vi "#459.vi"() -> ()   [LabVIEW 2017]
uses:
  user.lib/_NEVSTOP/Communicable State Machine(CSM)/Utility/_support/Periodic String Filter Level.ctl
  user.lib/_NEVSTOP/Communicable State Machine(CSM)/Utility/Periodic String Filter Setting.ctl
  user.lib/_NEVSTOP/Communicable State Machine(CSM)/AdvanceAPI/CSM - Revert Arguments-Safe String.vi
  user.lib/_NEVSTOP/Communicable State Machine(CSM)/_Shared/Trim Single-line Text.vi
  user.lib/_NEVSTOP/Communicable State Machine(CSM)/AdvanceAPI/CSM - Make String Arguments Safe.vi
  user.lib/_NEVSTOP/Communicable State Machine(CSM)/AdvanceAPI/CSM - Break Down Multiple States String.vi
  user.lib/_NEVSTOP/Communicable State Machine(CSM)/AdvanceAPI/CSM - Compact Multiple States.vi
  user.lib/_NEVSTOP/Communicable State Machine(CSM)/AdvanceAPI/CSM - Keywords.vi
  user.lib/_NEVSTOP/Communicable State Machine(CSM)/Communicable State Machine.lvlib
  user.lib/_NEVSTOP/Communicable State Machine(CSM)/addons/Watchdog/CSM Watchdog.lvlib
  user.lib/_NEVSTOP/Communicable State Machine(CSM)/addons/Logger/CSM File Logger.lvlib
  user.lib/_NEVSTOP/Communicable State Machine(CSM)/addons/Logger/CSM File Logger Limit.ctl
panel:
  out "State History 2":string
  in  "Exit":bool
  out "Waveform Chart":dbl(graph)
  out "Since Exiting(s)":dbl format="%.2f"
  out "LogInQ":i32
  out "State History":string
  out "log handling Speed(#/s)":dbl
  out "LogInQ changing Speed(#/s)":dbl
  out "Level":T1
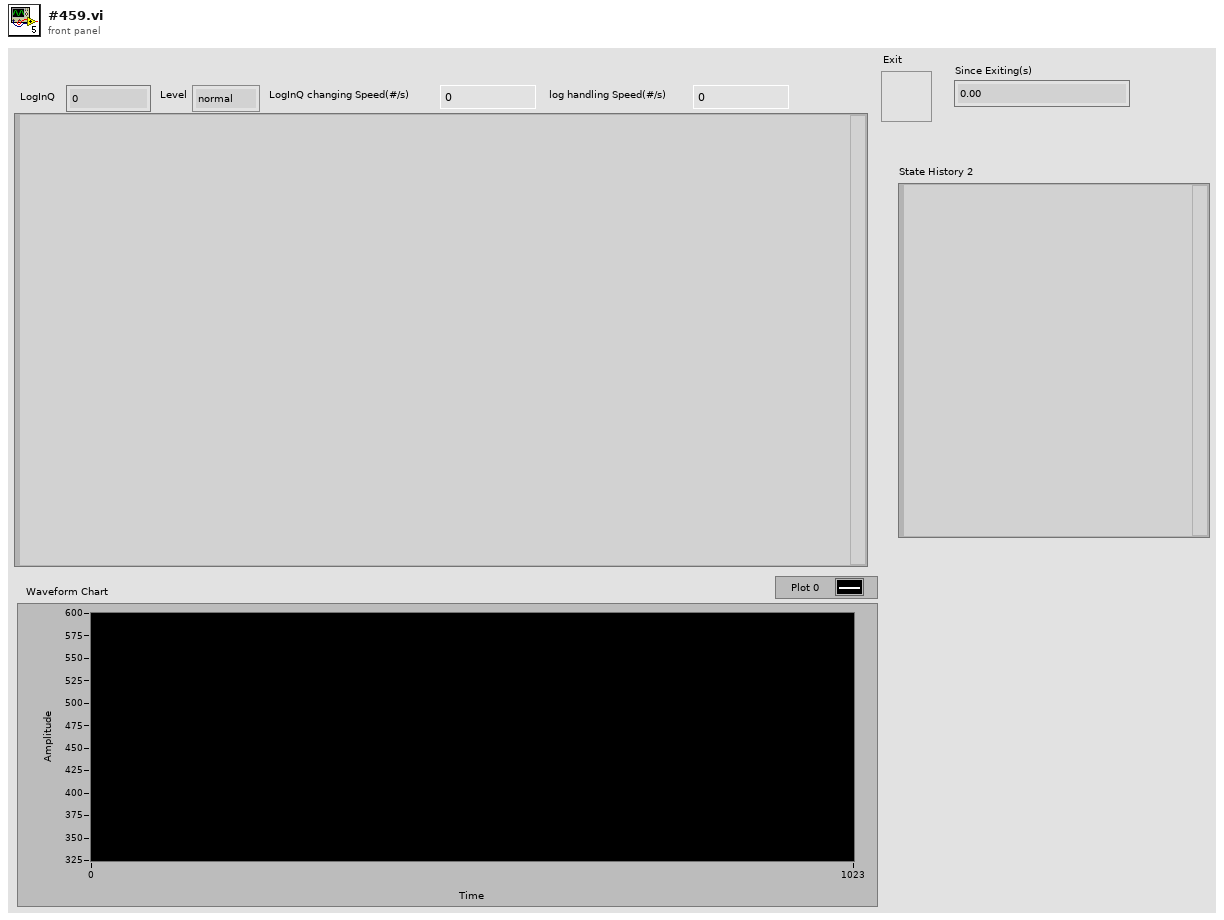
[diagram p1: front panel]
types:
  T1 = typedef "Communicable State Machine.lvlib/Periodic String Filter Level.ctl" = enum16{"normal", "L1", "L2", "L3", "L4"}
  T2 = typedef "CSM File Logger.lvlib/CSM File Logger Limit.ctl" = cluster{"file size (in bytes)":i64, "file num":i32}
  T3 = typedef "Communicable State Machine.lvlib/Periodic String Filter Setting.ctl" = cluster{"threashold(#/s)":dbl, "Check Peroid(s)":dbl}
  T4 = typedef "Communicable State Machine.lvlib/_CSM_GlobalLog_MSG.ctl" = cluster{"Name(\"\" to use uuid)":string, "Current State":string, "Arguments":string, "Source Message":T5, "Source Module":string, "Complete(T)/Start(F)":bool, "LogType":T6, "Time Stamp":timestamp}
  T5 = typedef "Communicable State Machine.lvlib/_CSM_Response Source Message.ctl" = cluster{"‘State":string, "’Arguments":string, "’Error":errorcluster}
  T6 = typedef "Communicable State Machine.lvlib/_CSM_GlobalLog_MSG_TYPE.ctl" = enum16{"User Log", "State Change", "Status", "Interrupt", "Register", "Unregister", "Error Log", "Module Created", "Module Destroyed"}
  T7 = enum32{"Invalid", "Standard", "Closed", "Hidden", "Minimized", "Maximized"}
  T8 = enum32{"invalid app kind", "Development System", "Run Time System", "Student Edition", "Embedded LabVIEW", "Evaluation", "Custom"}
  T9 = cluster{"Current VI Reference":refnum<vi>, "Close Panel on Exit?":bool}
  T10 = cluster{"Core":cluster{"Current VI Reference":refnum<vi>, "Close Panel on Exit?":bool}, "Your Boolean data":bool, "Your string data":string}
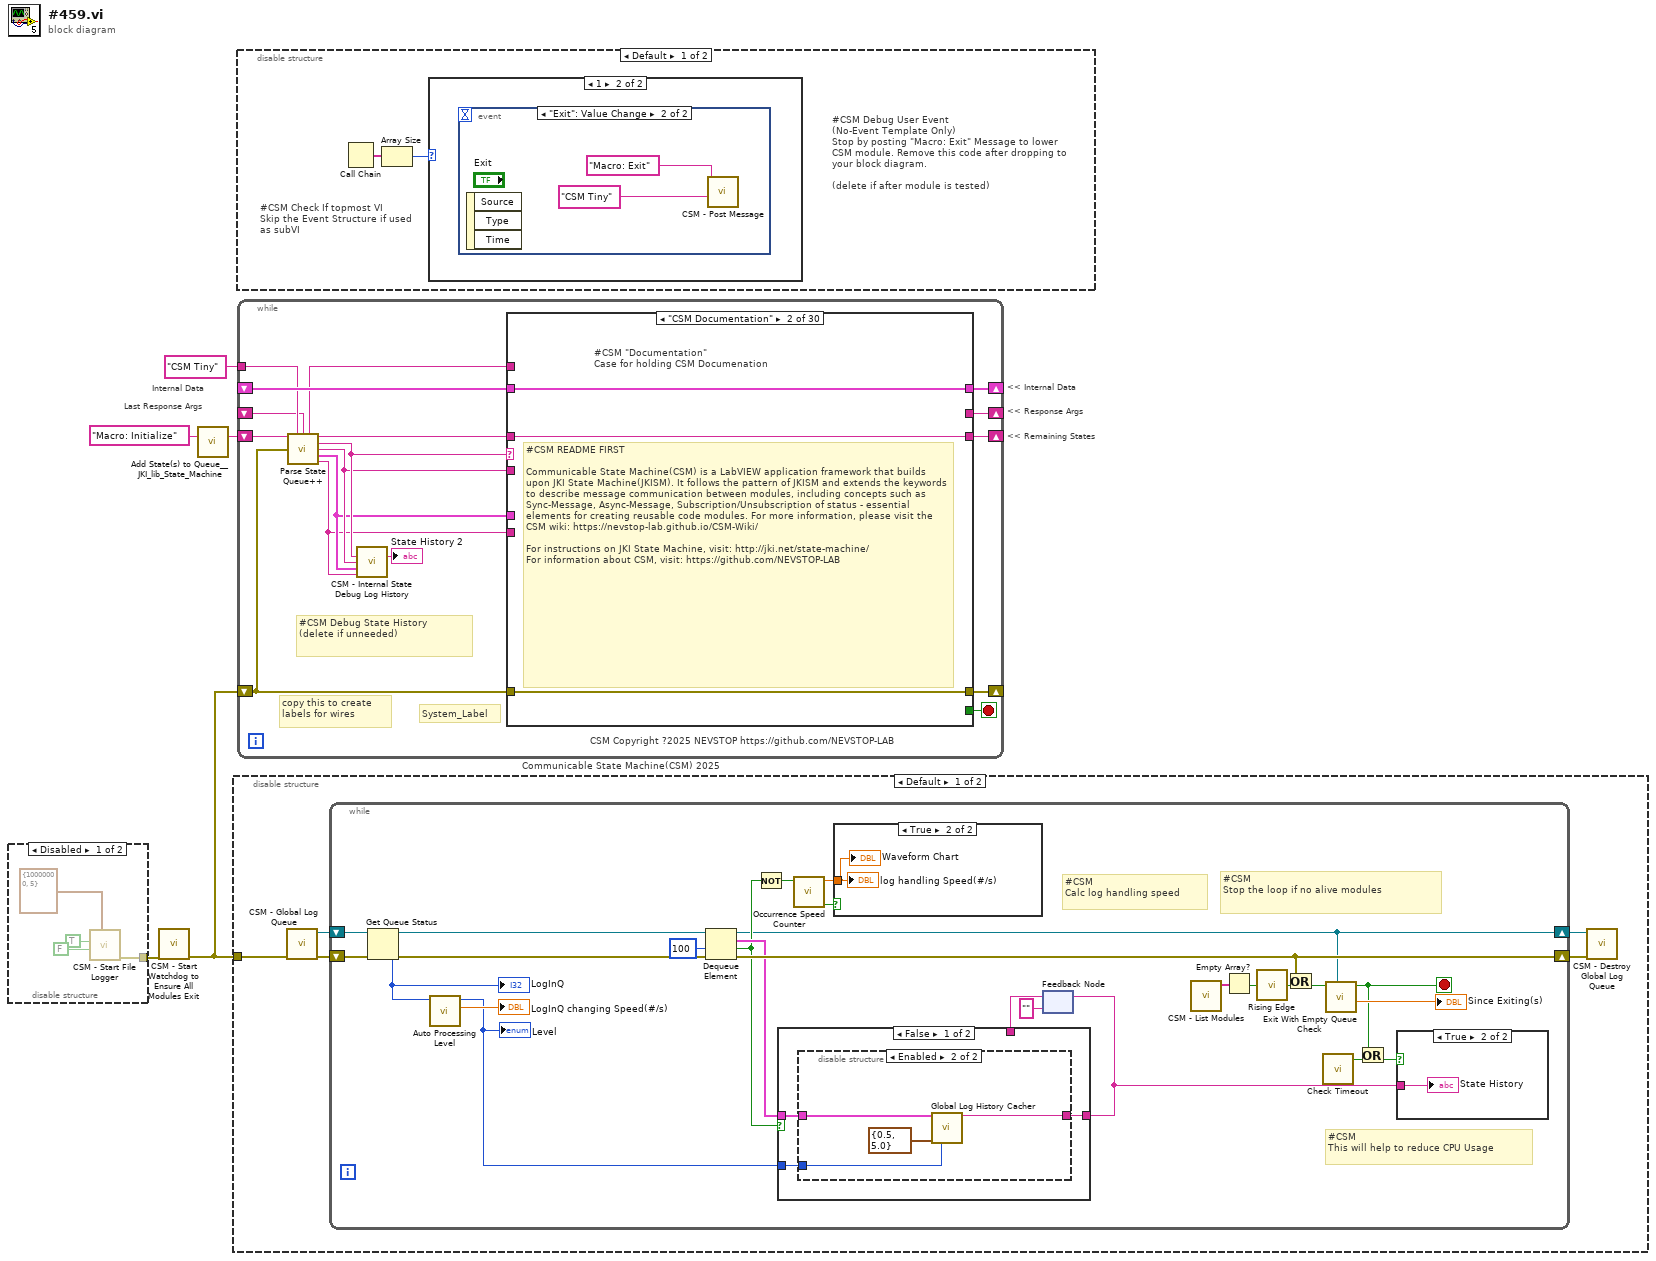
[diagram p0: block diagram]
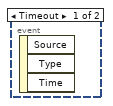
[diagram p3: hidden frame]
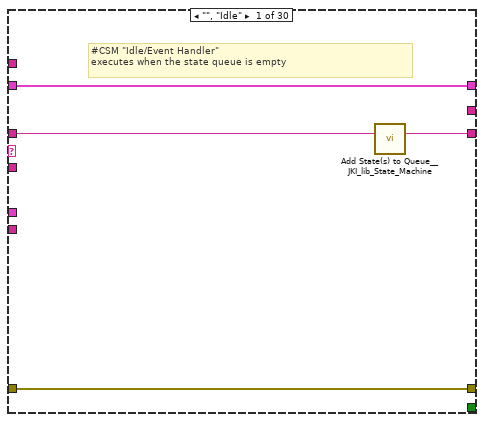
[diagram p5: hidden frame]
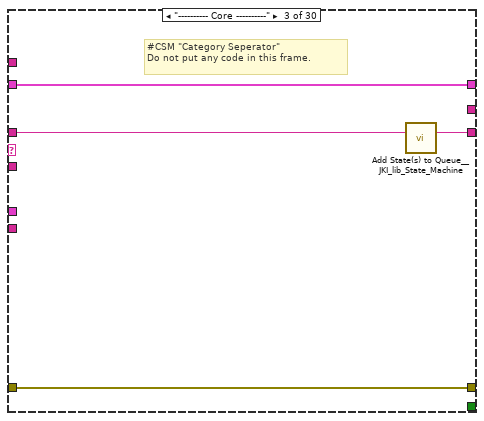
[diagram p6: hidden frame]
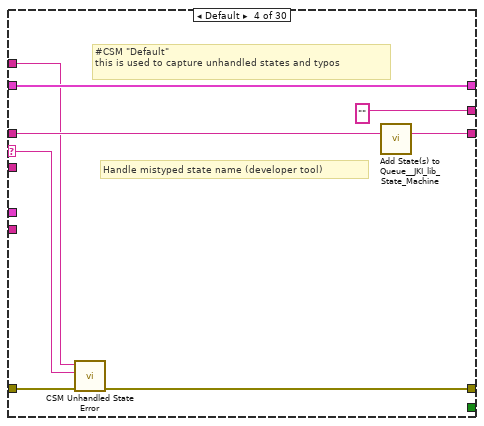
[diagram p7: hidden frame]
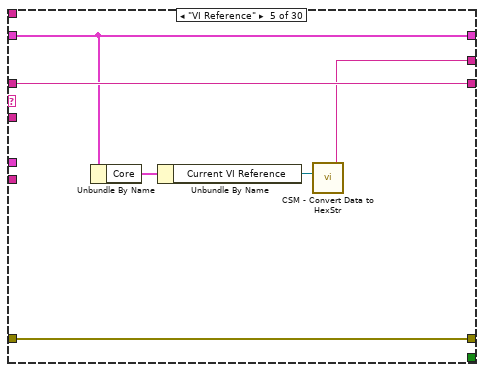
[diagram p8: hidden frame]
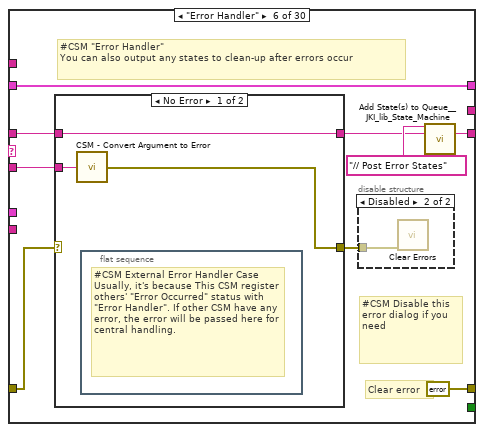
[diagram p9: hidden frame]
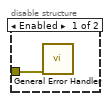
[diagram p10: hidden frame]
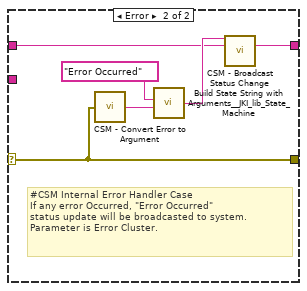
[diagram p11: hidden frame]
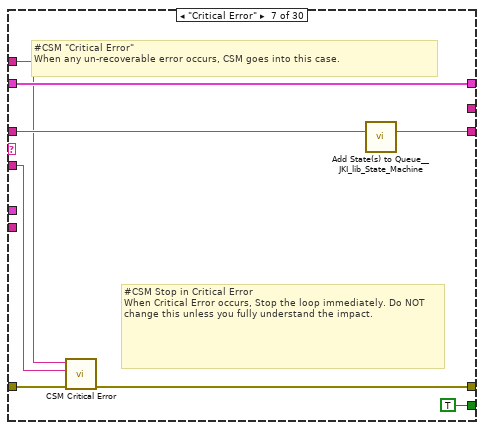
[diagram p12: hidden frame]
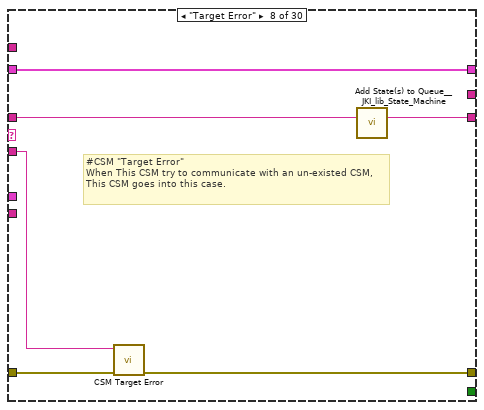
[diagram p13: hidden frame]
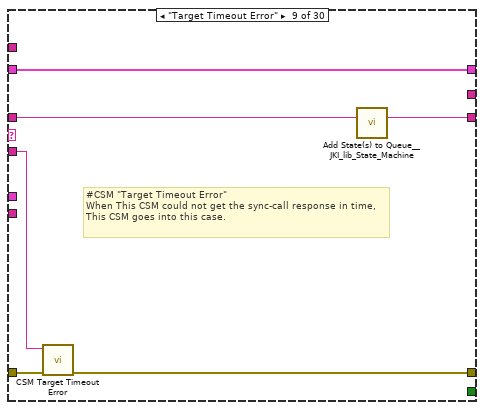
[diagram p14: hidden frame]
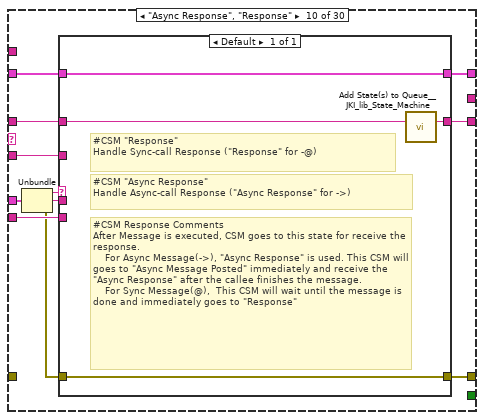
[diagram p15: hidden frame]
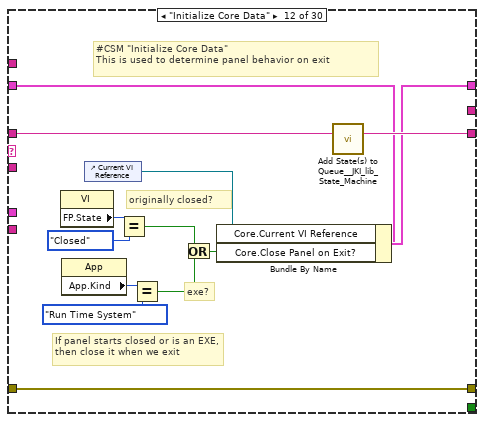
[diagram p17: hidden frame]
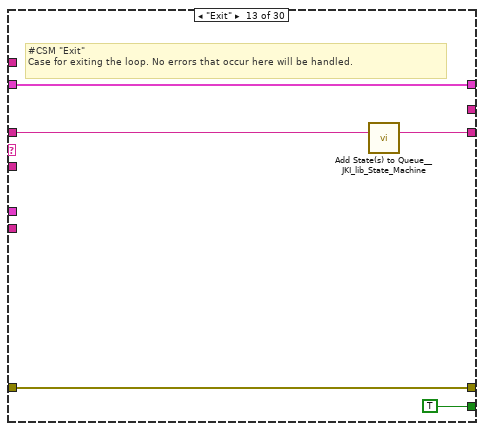
[diagram p18: hidden frame]
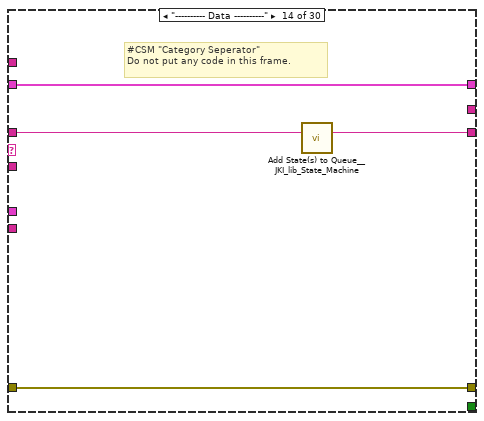
[diagram p19: hidden frame]
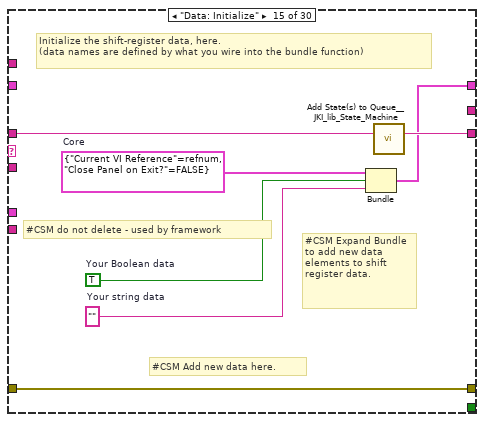
[diagram p20: hidden frame]
diagram:
  # "Last Response Args"
  # "Internal Data"
  # "<< Internal Data"
  # "<< Response Args"
  # "<< Remaining States"
  n1 = disable-structure shown="Disabled" {
    disable-tunnel: [w9 _] -> w5
    frame Disabled {
      n2 = call "CSM - Start File Logger.vi"("log limit"=T2 {"file size (in bytes)"=10000000, "file num"=5}, "WatchDog? (T)"=FALSE, "Exit When All Module Exist?(F)"=TRUE) -> ("Error out"=w9:errorcluster)  [unwired: 6 in, 2 out]
    }
    frame Enabled {
    }
  }
  n3 = call "CSM - Start Watchdog to Ensure All Modules Exit.vi"("error in (no error)"=w5) -> ("error out"=w1:errorcluster)  [unwired: 10 in]
  n4 = call <vilib>:"Add State(s) to Queue__JKI_lib_State_Machine.vi"("State(s) in (\"\")"="Macro: Initialize" ("Init State(\"Macro: Initialize\")")) -> ("States Out"=w2:string)  [unwired: 14 in]
  n5 = disable-structure shown="Default" {
    disable-tunnel: w1 -> [w10 _]
    frame condition #0 (active) {
      n6 = call "CSM - Global Log Queue.vi"("Error in"=w10) -> ("Error out"=w13:errorcluster, "GlobalEvent Queue"=w11:refnum<queue>)  [unwired: 9 in]
      n7 = while {
        shift-right: [w39] -> w14
        shift-left: w13 -> [w36]
        shift-right: [w27] -> w12
        shift-left: w11 -> [w40]
        stop <- w20 stop-if-true
        # "#CSM\nCalc log handling speed"
        # "#CSM\nStop the loop if no alive modules"
        # "#CSM\nThis will help to reduce CPU Usage"
        n8 = Get Queue Status(queue=w40, error in (no error)=w36) -> (queue out=w38:refnum<queue>, error out=w37:errorcluster, # elements in queue=w23:i32)  [unwired: 1 in, 5 out]
        "LogInQ" <- w23
        n9 = call "Auto Processing Level.vi"("#Left In Q"=w23) -> ("LogInQ changing Speed(#/s)"=→"LogInQ changing Speed(#/s)":dbl, "Level"=w22:T1)  [unwired: 8 in, 1 out]
        "Level" <- w22
        n10 = Dequeue Element(queue=w38, timeout in ms (-1)=100, error in (no error)=w37) -> (queue out=w27:refnum<queue>, element=w35:T4, timed out?=w29:bool, error out=w39:errorcluster)
        n11 = Not(x=w29) -> (.not. x?=w28:bool)
        n12 = call "Occurrence Speed Counter.vi"("Occured?(T)"=w28) -> ("New?"=w18:bool, "Speed(#/s)"=w19:dbl)  [unwired: 8 in, 1 out]
        n13 = case shown="True" w18 {
          tunnel: w19 -> [_ w41]
          frame False {
          }
          frame True {
            "log handling Speed(#/s)" <- w41
            "Waveform Chart" <- w41
          }
        }
        n14 = feedback #1("" ("String Cache")) -> (w31:string)
        n15 = case shown="False" w29 {
          tunnel: w35 -> [w44 _]
          tunnel: [w43 w52] -> w32
          tunnel: w31 -> [_ w52]
          tunnel: w22 -> [w42 _]
          frame False {
            n16 = disable-structure shown="Enabled" {
              disable-tunnel: w44 -> [w47 w50]
              disable-tunnel: [w45 w51] -> w43
              disable-tunnel: w42 -> [_ w49]
              frame Disabled {
                # "#CSM \nno periodical filter"
                n17 = call "Global Log To String(Source Time).vi"("Log"=w47) -> ("Log String"=w46:string)  [unwired: 9 in]
                n18 = call "String History Cacher.vi"("String"=w46) -> ("String Cache"=w45:string)  [unwired: 10 in]
              }
              frame Enabled {
                n19 = call "Global Log History Cacher.vi"("Cross CSM Data"=w50, "Settings"=T3 {"threashold(#/s)"=0.5, "Check Peroid(s)"=5.0}, "Level(Normal)"=w49) -> ("String Cache"=w51:string)  [unwired: 12 in]
              }
            }
          }
          frame True {
          }
        }
        n20 = feedback-in #1(w32) -> ()
        n21 = call "CSM - List Modules.vi"() -> ("Module Names"=w15:string[])  [unwired: 10 in, 1 out]
        n22 = Empty Array?(array=w15) -> (empty?=w17:bool)
        n23 = call "Rising Edge.vi"("signal"=w17) -> ("rising edge"=w16:bool)
        n24 = Or(x=w39, y=w16) -> (x .or. y?=w25:bool)
        n25 = call "Check Timeout.vi"() -> ("Timeout"=w33:bool)  [unwired: 8 in]
        n26 = call "Exit With Empty Queue Check.vi"("queue"=w27, "Stop"=w25) -> ("Since Exiting(s)"=→"Since Exiting(s)":dbl, "exit"=w20:bool)  [unwired: 8 in]
        n27 = Or(x=w20, y=w33) -> (x .or. y?=w26:bool)
        n28 = case shown="True" w26 {
          tunnel: w32 -> [_ w53]
          frame False {
          }
          frame True {
            "State History" <- w53
          }
        }
      }
      n29 = call "CSM - Destroy Global Log Queue.vi"("Error in"=w14, "CreatedQueue"=w12) -> ()  [unwired: 9 in, 1 out]
    }
    frame condition #1 {
    }
  }
  n30 = disable-structure shown="Default" {
    frame condition #0 (active) {
      # "#CSM Check If topmost VI\nSkip the Event Structure if used as subVI"
      # "#CSM Debug User Event\n(No-Event Template Only)\nStop by posting \"Macro: Exit\" Message to lower CSM module. Remove this code after dropping to your block diagram. \n\n(delete if after module is tested)"
      n31 = Call Chain() -> (call chain=w55:string[])
      n32 = Array Size(array=w55) -> (size(s)=w54:i32)
      n33 = case shown="1" w54 {
        frame Default {
        }
        frame 1 {
          n34 = event shown="[1] \"Exit\": Value Change" {
            selector: _ -> [_ _]
            dyn-events: _ -> [_ _]
            timeout: _ -> [_ _]
            event Timeout {
              n35 = event-data() -> ()  [unwired: 1 in, 3 out]
            }
            event "Exit": Value Change {
              n36 = event-data() -> ()  [unwired: 1 in, 3 out]
              n37 = call "CSM - Post Message.vi"("Target Module"="CSM Tiny" ("Name(\"\" to use uuid)"), "State"="Macro: Exit" ("States")) -> ()  [unwired: 9 in, 1 out]
            }
          }
        }
      }
    }
    frame condition #1 {
    }
  }
  n38 = while "Communicable State Machine(CSM) 2025" {
    shift-right: [w69] -> _
    shift-left: _ -> [w68]
    shift-right: [w72] -> _
    shift-left: w1 -> [w67]
    shift-right: [w71] -> _
    shift-left: w2 -> [w73]
    tunnel: "CSM Tiny" ("Name(\"\" to use uuid)") -> [w65]
    shift-right: [w66] -> _
    shift-left: _ -> [w59]
    stop <- w70 stop-if-true
    # "#CSM Debug State History\n(delete if unneeded)"
    # "copy this to create labels for wires"
    # "System_Label"
    # "CSM Copyright ?2025 NEVSTOP https://github.com/NEVSTOP-LAB"
    n39 = call "Parse State Queue++.vi"("State Queue"=w73, "Name(\"\" to use uuid)"=w65, "Response Arguments"=w59, "Previous Error"=w67) -> ("Name Used"=w60:string, "Remaining States"=w74:string, "Current State"=w64:string, "Arguments"=w63:string, ">> Response Source Message >>"=w62:T5, ">> Source CSM >>"=w61:string)  [unwired: 6 in]
    n40 = call "CSM - Internal State Debug Log History.vi"("State"=w64, "Arguments (\"\")"=w63, ">> Response Source Message >>"=w62, "Source (\"\")"=w61) -> ("Debug Log"=→"State History 2":string)  [unwired: 11 in]
    n41 = case shown="\"CSM Documentation\"" w64 {
      selector: w64 -> [_ _ _ w88 _ _ _ _ _ _ _ _ _ _ _ _ _ _ _ _ _ _ _ _ _ _ _ _ _ _]
      tunnel: w74 -> [w75 w80 w85 w92 w98 w104 w125 w131 w137 w145 w156 w170 w175 w179 w186 w188 w195 w199 w203 w209 w224 w293 w298 w305 w307 w311 w316 w323 w327 w331]
      tunnel: w63 -> [_ _ _ _ _ w103 w121 w130 w135 w144 _ _ _ _ _ _ _ _ _ w204 w218 _ _ _ _ _ w314 _ _ _]
      tunnel: w68 -> [w76 w79 w82 w90 w97 w107 w126 w132 w138 w147 w155 w163 w173 w176 _ w187 w190 w196 w201 w207 w220 w290 w295 w302 w306 w310 w315 w320 w324 w328]
      tunnel: [w77 w81 w83 w86 w99 errorcluster {"status"=FALSE, "code"=0, "source"=""} ("error out") w122 w128 w134 w150 w157 w167 w172 w177 w183 w189 w191 w197 w200 w205 w221 w291 w296 w303 w308 w312 w317 w321 w325 w329] -> w72
      tunnel: w67 -> [w77 w81 w83 w93 w99 w105 w127 w129 w136 _ w157 w167 w172 w177 w183 w189 w192 w197 w200 w206 w222 w291 w296 w303 w308 w312 w317 w321 w325 w329]
      tunnel: [w78 w80 w84 w91 w98 w100 w124 w133 w139 w146 w156 w169 w174 w178 w185 w188 w194 w198 w202 w208 w223 w292 w297 w304 w307 w311 w316 w322 w326 w330] -> w71
      tunnel: [_ _ _ _ _ _ TRUE _ _ _ _ _ TRUE _ _ _ _ _ _ _ _ _ _ _ _ _ _ _ _ _] -> w70
      tunnel: [w76 w79 w82 w90 w97 w107 w126 w132 w138 w148 w155 w168 w173 w176 w184 w187 w190 w196 w201 w207 w220 w290 w295 w302 w306 w310 w315 w320 w324 w328] -> w69
      tunnel: w61 -> [_ _ _ _ _ _ _ _ _ w142 _ _ _ _ _ _ _ _ _ _ _ _ _ _ _ _ _ _ _ _]
      tunnel: w62 -> [_ _ _ _ _ _ _ _ _ w149 _ _ _ _ _ _ _ _ _ _ _ _ _ _ _ _ _ _ _ _]
      tunnel: [_ _ _ "" w94 _ _ _ _ _ _ _ _ _ _ _ _ _ _ _ _ _ _ _ _ "API1 Response" w313 _ _ _] -> w66
      tunnel: w60 -> [_ _ _ w87 _ _ w120 _ _ _ _ _ _ _ _ _ _ _ _ _ _ _ _ _ _ _ _ _ _ _]
      frame "", "Idle" {
        # "#CSM \"Idle/Event Handler\"\nexecutes when the state queue is empty"
        n42 = call <vilib>:"Add State(s) to Queue__JKI_lib_State_Machine.vi"("State(s) in (\"\")"=w75) -> ("States Out"=w78:string)  [unwired: 14 in]
      }
      frame "CSM Documentation" {
        # "#CSM README FIRST\n\nCommunicable State Machine(CSM) is a LabVIEW application framework that builds upon JKI State Machine(JKISM). It follows the pattern of JKISM and extends the keywords to describe message communication between modules, including concepts such as Sync-Message, Async-Message, Subscription/Unsubscription of status - essential elements for creating reusable code modules. For more information, please visit the CSM wiki: https://nevstop-lab.github.io/CSM-Wiki/\n\nFor instructions on JKI State Machine, visit: http://jki.net/state-machine/\nFor information about CSM, visit: https://github.com/NEVSTOP-LAB"
        # "#CSM \"Documentation\"\nCase for holding CSM Documenation"
      }
      frame "---------- Core ----------" {
        # "#CSM \"Category Seperator\"\nDo not put any code in this frame."
        n43 = call <vilib>:"Add State(s) to Queue__JKI_lib_State_Machine.vi"("State(s) in (\"\")"=w85) -> ("States Out"=w84:string)  [unwired: 14 in]
      }
      frame Default {
        # "#CSM \"Default\"\nthis is used to capture unhandled states and typos"
        # "Handle mistyped state name (developer tool)"
        n44 = call "CSM Unhandled State Error.vi"("error in (no error)"=w93, "Current State"=w88, "CSM Name"=w87) -> ("error out"=w86:errorcluster)  [unwired: 8 in]
        n45 = call <vilib>:"Add State(s) to Queue__JKI_lib_State_Machine.vi"("State(s) in (\"\")"=w92) -> ("States Out"=w91:string)  [unwired: 14 in]
      }
      frame "VI Reference" {
        n46 = Unbundle By Name(w97) -> ("Core"=w96:T9)
        n47 = Unbundle By Name(w96) -> ("Current VI Reference"=w95:refnum<vi>)
        n48 = call "CSM - Convert Data to HexStr.vi"("Variant"=w95) -> ("HEX String (0-9,A-F)"=w94:string)  [unwired: 8 in]
      }
      frame "Error Handler" {
        # "#CSM Disable this error dialog if you need"
        # "#CSM \"Error Handler\"\nYou can also output any states to clean-up after errors occur"
        # "Clear error"
        n49 = case shown="No Error" w105 {
          selector: w105 -> [_ w114]
          tunnel: [w113 w116] -> w101
          tunnel: w104 -> [w113 w115]
          tunnel: w103 -> [w112 _]
          tunnel: [w111 w114] -> w106
          frame No Error {
            n50 = call "CSM - Convert Argument to Error.vi"("Argument"=w112) -> ("error"=w111:errorcluster)  [unwired: 4 in]
            n51 = flat-sequence {
              frame #0 {
                # "#CSM External Error Handler Case\nUsually, it's because This CSM register others' \"Error Occurred\" status with \"Error Handler\". If other CSM have any error, the error will be passed here for central handling."
              }
            }
          }
          frame Error {
            # "#CSM Internal Error Handler Case \nIf any error Occurred, \"Error Occurred\" \nstatus update will be broadcasted to system.\nParameter is Error Cluster."
            n52 = call "CSM - Convert Error to Argument.vi"("error"=w114) -> ("Argument"=w118:string)  [unwired: 4 in]
            n53 = call <vilib>:"Build State String with Arguments__JKI_lib_State_Machine.vi"("Arguments (\"\")"=w118, "State"="Error Occurred" ("Status with Arguments")) -> ("State with Arguments"=w117:string)  [unwired: 4 in]
            n54 = call "CSM - Broadcast Status Change.vi"("Status with Arguments"=w117, "State Queue"=w115) -> ("Remaining States"=w116:string)  [unwired: 13 in]
          }
        }
        n55 = disable-structure shown="Disabled" {
          disable-tunnel: w106 -> [w109 w110]
          frame Enabled {
            n56 = call <vilib>:"General Error Handler.vi"("error in (no error)"=w109) -> ()  [unwired: 10 in, 5 out]
          }
          frame Disabled {
            n57 = call <vilib>:"Clear Errors.vi"("error in (no error)"=w110) -> ()  [unwired: 5 in, 2 out]
          }
        }
        n58 = call <vilib>:"Add State(s) to Queue__JKI_lib_State_Machine.vi"("State(s) in Front (\"\")"="// Post Error States", "State(s) in (\"\")"=w101) -> ("States Out"=w100:string)  [unwired: 13 in]
      }
      frame "Critical Error" {
        # "#CSM Stop in Critical Error\nWhen Critical Error occurs, Stop the loop immediately. Do NOT change this unless you fully understand the impact."
        # "#CSM \"Critical Error\"\nWhen any un-recoverable error occurs, CSM goes into this case."
        n59 = call "CSM Critical Error.vi"("error in (no error)"=w127, "Arugments(as Reason)"=w121, "CSM Name"=w120) -> ("error out"=w122:errorcluster)  [unwired: 8 in]
        n60 = call <vilib>:"Add State(s) to Queue__JKI_lib_State_Machine.vi"("State(s) in (\"\")"=w125) -> ("States Out"=w124:string)  [unwired: 14 in]
      }
      frame "Target Error" {
        # "#CSM \"Target Error\"\nWhen This CSM try to communicate with an un-existed CSM, This CSM goes into this case."
        n61 = call "CSM Target Error.vi"("error in (no error)"=w129, "Arguments(as CSM Name)"=w130) -> ("error out"=w128:errorcluster)  [unwired: 9 in]
        n62 = call <vilib>:"Add State(s) to Queue__JKI_lib_State_Machine.vi"("State(s) in (\"\")"=w131) -> ("States Out"=w133:string)  [unwired: 14 in]
      }
      frame "Target Timeout Error" {
        # "#CSM \"Target Timeout Error\"\nWhen This CSM could not get the sync-call response in time, This CSM goes into this case."
        n63 = call "CSM Target Timeout Error.vi"("error in (no error)"=w136, "Arguments(as CSM Name)"=w135) -> ("error out"=w134:errorcluster)  [unwired: 9 in]
        n64 = call <vilib>:"Add State(s) to Queue__JKI_lib_State_Machine.vi"("State(s) in (\"\")"=w137) -> ("States Out"=w139:string)  [unwired: 14 in]
      }
      frame "Async Response", "Response" {
        n65 = Unbundle(w149) -> ("‘State"=w143:string, "’Arguments"=w141:string, "’Error"=w140:errorcluster)
        n66 = case shown="Default" w143 {
          tunnel: [w154] -> w150
          tunnel: w140 -> [w154]
          tunnel: [w153] -> w148
          tunnel: w147 -> [w153]
          tunnel: [w151] -> w146
          tunnel: w145 -> [w152]
          tunnel: w144 -> [_]
          tunnel: w142 -> [_]
          tunnel: w141 -> [_]
          frame Default {
            # "#CSM Response Comments\nAfter Message is executed, CSM goes to this state for receive the response.\n    For Async Message(->), \"Async Response\" is used. This CSM will goes to \"Async Message Posted\" immediately and receive the \"Async Response\" after the callee finishes the message.\n    For Sync Message(@),  This CSM will wait until the message is done and immediately goes to \"Response\""
            # "#CSM \"Async Response\"\nHandle Async-call Response (\"Async Response\" for ->)"
            # "#CSM \"Response\"\nHandle Sync-call Response (\"Response\" for -@)"
            n67 = call <vilib>:"Add State(s) to Queue__JKI_lib_State_Machine.vi"("State(s) in (\"\")"=w152) -> ("States Out"=w151:string)  [unwired: 14 in]
          }
        }
      }
      frame "Async Message Posted" {
        # "#CSM \"Async Message Posted\"\nAfter Async Message is posted (-> or ->| ), CSM goes to this state for post-action.\nYou can use Argument - State to tell which Async Message is called."
      }
      frame "Initialize Core Data" {
        # "#CSM \"Initialize Core Data\"\nThis is used to determine panel behavior on exit"
        # "originally closed?"
        # "exe?"
        # "If panel starts closed or is an EXE, then close it when we exit"
        n68 = property class="VI"() -> ("FP.State"=w160:T7)  [unwired: 2 in, 2 out]
        n69 = property class="App"() -> ("App.Kind"=w166:T8)  [unwired: 2 in, 2 out]
        n70 = control-ref of="Current VI Reference"() -> (w161:refnum<vi>)
        n71 = Equal?(x=w160, y=T7."Closed" ("Front Panel Window:State")) -> (x = y?=w158:bool)
        n72 = Equal?(x=w166, y=T8."Run Time System" ("Application:Kind")) -> (x = y?=w164:bool)
        n73 = Or(x=w158, y=w164) -> (x .or. y?=w162:bool)
        n74 = Bundle By Name(cluster=w163, "Core.Current VI Reference"=w161, "Core.Close Panel on Exit?"=w162) -> (w168:T10)
        n75 = call <vilib>:"Add State(s) to Queue__JKI_lib_State_Machine.vi"("State(s) in (\"\")"=w170) -> ("States Out"=w169:string)  [unwired: 14 in]
      }
      frame "Exit" {
        # "#CSM \"Exit\"\nCase for exiting the loop. No errors that occur here will be handled."
        n76 = call <vilib>:"Add State(s) to Queue__JKI_lib_State_Machine.vi"("State(s) in (\"\")"=w175) -> ("States Out"=w174:string)  [unwired: 14 in]
      }
      frame "---------- Data ----------" {
        # "#CSM \"Category Seperator\"\nDo not put any code in this frame."
        n77 = call <vilib>:"Add State(s) to Queue__JKI_lib_State_Machine.vi"("State(s) in (\"\")"=w179) -> ("States Out"=w178:string)  [unwired: 14 in]
      }
      frame "Data: Initialize" {
        w180 = T9 {"Current VI Reference"=refnum, "Close Panel on Exit?"=FALSE}  # Core
        w182 = TRUE  # Your Boolean data
        w181 = ""  # Your string data
        # "#CSM do not delete - used by framework"
        # "#CSM Expand Bundle to add new data elements to shift register data."
        # "#CSM Add new data here."
        # "Initialize the shift-register data, here.\n(data names are defined by what you wire into the bundle function)"
        n78 = Bundle("Core"=w180, "Your Boolean data"=w182, "Your string data"=w181) -> (w184:T10)  [unwired: 1 in]
        n79 = call <vilib>:"Add State(s) to Queue__JKI_lib_State_Machine.vi"("State(s) in (\"\")"=w186) -> ("States Out"=w185:string)  [unwired: 14 in]
      }
      frame "Data: Update Indicators" {
      }
      frame "Data: Cleanup" {
        # "Cleanup any data and references, here.\n(this is called automatically, by the Macro: Exit)"
        n80 = Unbundle By Name(w190) -> ("Core.Current VI Reference"=w193:refnum<vi>)
        n81 = Close Reference(reference=w193, error in (no error)=w192) -> (error out=w191:errorcluster)
        n82 = call <vilib>:"Add State(s) to Queue__JKI_lib_State_Machine.vi"("State(s) in (\"\")"=w195) -> ("States Out"=w194:string)  [unwired: 14 in]
      }
      frame "---------- UI ----------" {
        # "#CSM \"Category Seperator\"\nDo not put any code in this frame."
        n83 = call <vilib>:"Add State(s) to Queue__JKI_lib_State_Machine.vi"("State(s) in (\"\")"=w199) -> ("States Out"=w198:string)  [unwired: 14 in]
      }
      frame "UI: Initialize" {
        # "#CSM \"UI: Initialize\"\nInitialize the User Interface, here.\n(this is called automatically, by the Macro: Init)"
        n84 = call <vilib>:"Add State(s) to Queue__JKI_lib_State_Machine.vi"("State(s) in (\"\")"=w203) -> ("States Out"=w202:string)  [unwired: 14 in]
      }
      frame "UI: Cursor Set" {
        # "#CSM \"UI: Cursor Set\"\nSet and Unset Cursor Busy.\n(Usage: \"UI: Cursor Set >> Busy|Idle\")"
        # "Argument"
        n85 = disable-structure shown="TARGET_TYPE!=Windows" {
          disable-tunnel: w206 -> [w212 w217]
          disable-tunnel: [w211 w217] -> w205
          disable-tunnel: w204 -> [w210 _]
          frame condition #0 (active) {
            n86 = case shown="\"Idle\", Default" w210 {
              tunnel: w212 -> [w214 w216]
              tunnel: [w213 w215] -> w211
              frame "Idle", Default {
                n87 = call <vilib>:"Unset Busy.vi"("error in (no error)"=w214) -> ("error out"=w213:errorcluster)  [unwired: 10 in]
              }
              frame "Busy" {
                n88 = call <vilib>:"Set Busy.vi"("error in (no error)"=w216) -> ("error out"=w215:errorcluster)  [unwired: 9 in, 1 out]
              }
            }
          }
          frame condition #1 {
          }
        }
        n89 = call <vilib>:"Add State(s) to Queue__JKI_lib_State_Machine.vi"("State(s) in (\"\")"=w209) -> ("States Out"=w208:string)  [unwired: 14 in]
      }
      frame "UI: Front Panel State" {
        # "#CSM \"UI: Front Panel State\"\nSet Front Panel Open or Closed\n(Usage: \"UI: Front Panel State >> Open|Close\")"
        # "Argument"
        n90 = Unbundle By Name(w220) -> ("Core.Current VI Reference"=w219:refnum<vi>)
        n91 = call <vilib>:"Add State(s) to Queue__JKI_lib_State_Machine.vi"("State(s) in (\"\")"=w224) -> ("States Out"=w223:string)  [unwired: 14 in]
        n92 = case shown="\"Close\", \"Closed\"" w218 {
          tunnel: w222 -> [w230 w245 w256 w269 w282]
          tunnel: [w232 w246 w258 w271 w284] -> w221
          tunnel: w219 -> [w231 w243 w257 w270 w283]
          frame "Open", "Standard", Default {
            w225 = T7."Standard" ("State")
            n93 = property class="VI"(reference=w231, error in=w230) -> (reference out=w228:refnum<vi>, error out=w229:errorcluster, "FP.State"=w227:T7)
            n94 = Not Equal?(x=w227, y=w225) -> (x != y?=w226:bool)
            n95 = case shown="True" w226 {
              tunnel: [w236 w238] -> w232
              tunnel: w229 -> [w235 w238]
              tunnel: w228 -> [w234 _]
              tunnel: w225 -> [w233 _]
              frame True {
                n96 = invoke class="VI" method="FP.Open"(reference=w234, error in=w235, "Activate"=TRUE, "State"=w233) -> (error out=w236:errorcluster)  [unwired: 1 in, 4 out]
              }
              frame False {
              }
            }
          }
          frame "Close", "Closed" {
            n97 = property class="VI"(reference=w243, error in=w245) -> (reference out=w242:refnum<vi>, error out=w244:errorcluster, "FP.State"=w240:T7)
            n98 = Not Equal?(x=w240, y=T7."Closed" ("Front Panel Window:State")) -> (x != y?=w239:bool)
            n99 = case shown="False" w239 {
              tunnel: [w247 w250] -> w246
              tunnel: w244 -> [w247 w249]
              tunnel: w242 -> [_ w248]
              frame False {
              }
              frame True {
                n100 = invoke class="VI" method="FP.Close"(reference=w248, error in=w249) -> (error out=w250:errorcluster)  [unwired: 1 in, 2 out]
              }
            }
          }
          frame "Hidden", "Hide" {
            w251 = T7."Hidden" ("State")
            n101 = property class="VI"(reference=w257, error in=w256) -> (reference out=w254:refnum<vi>, error out=w255:errorcluster, "FP.State"=w253:T7)
            n102 = Not Equal?(x=w253, y=w251) -> (x != y?=w252:bool)
            n103 = case shown="True" w252 {
              tunnel: [w262 w263] -> w258
              tunnel: w255 -> [w261 w263]
              tunnel: w254 -> [w260 _]
              tunnel: w251 -> [w259 _]
              frame True {
                n104 = invoke class="VI" method="FP.Open"(reference=w260, error in=w261, "State"=w259) -> (error out=w262:errorcluster)  [unwired: 2 in, 4 out]
              }
              frame False {
              }
            }
          }
          frame "Minimize", "Minimized" {
            w264 = T7."Minimized" ("State")
            n105 = property class="VI"(reference=w270, error in=w269) -> (reference out=w267:refnum<vi>, error out=w268:errorcluster, "FP.State"=w266:T7)
            n106 = Not Equal?(x=w266, y=w264) -> (x != y?=w265:bool)
            n107 = case shown="True" w265 {
              tunnel: [w275 w276] -> w271
              tunnel: w268 -> [w274 w276]
              tunnel: w267 -> [w273 _]
              tunnel: w264 -> [w272 _]
              frame True {
                n108 = invoke class="VI" method="FP.Open"(reference=w273, error in=w274, "State"=w272) -> (error out=w275:errorcluster)  [unwired: 2 in, 4 out]
              }
              frame False {
              }
            }
          }
          frame "Maximize", "Maximized" {
            w277 = T7."Maximized" ("State")
            n109 = property class="VI"(reference=w283, error in=w282) -> (reference out=w280:refnum<vi>, error out=w281:errorcluster, "FP.State"=w279:T7)
            n110 = Not Equal?(x=w279, y=w277) -> (x != y?=w278:bool)
            n111 = case shown="True" w278 {
              tunnel: [w288 w289] -> w284
              tunnel: w281 -> [w287 w289]
              tunnel: w280 -> [w286 _]
              tunnel: w277 -> [w285 _]
              frame True {
                n112 = invoke class="VI" method="FP.Open"(reference=w286, error in=w287, "State"=w285) -> (error out=w288:errorcluster)  [unwired: 2 in, 4 out]
              }
              frame False {
              }
            }
          }
        }
      }
      frame "---------- Macro ----------" {
        # "#CSM \"Category Seperator\"\nDo not put any code in this frame."
        n113 = call <vilib>:"Add State(s) to Queue__JKI_lib_State_Machine.vi"("State(s) in (\"\")"=w293) -> ("States Out"=w292:string)  [unwired: 14 in]
      }
      frame "Macro: Initialize" {
        # "#CSM \"Macro: Initialize\"\nInitialization Macro (This is called once, when the VI starts)"
        n114 = call <vilib>:"Add State(s) to Queue__JKI_lib_State_Machine.vi"("State(s) in Front (\"\")"="Data: Initialize\nInitialize Core Data\nData: Update Indicators", "State(s) in (\"\")"=w298) -> ("States Out"=w297:string)  [unwired: 13 in]
      }
      frame "Macro: Exit" {
        # "#CSM \"Macro: Exit\"\nExit Macro (This is called once, when the VI exits)"
        n115 = call <vilib>:"Add State(s) to Queue__JKI_lib_State_Machine.vi"("State(s) in Front (\"\")"="//Exit Sub-Modules ", "State(s) at Back (\"\")"="Data: Cleanup\nExit") -> ("States Out"=w300:string)  [unwired: 13 in]
        n116 = call <vilib>:"Add State(s) to Queue__JKI_lib_State_Machine.vi"("State(s) in Front (\"\")"=w300, "State(s) in (\"\")"=w305) -> ("States Out"=w304:string)  [unwired: 13 in]
      }
      frame "---------- API ----------" {
        # "#CSM \"Category Seperator\"\nDo not put any code in this frame."
      }
      frame "API: API1" {
        # "#CSM API Example\nCopy/Rename this case for your own API"
        # "#CSM Response\nConnect this to return the response of your API"
        # "#CSM >> Msg/Rep's CSM >>\nIf you need to tell who triggered this state , use this string. If it's this case itself, this string is \"\"."
        # "#CSM >> Arguments >>\nDeal with the parameter if any"
      }
      frame "API: API2" {
        # "#CSM API Example\nCopy/Rename this case for your own API"
        # "unpack Hex String  to Variant\nif complex parameter is needed."
        n117 = call "CSM - Convert HexStr to Data.vi"("HEX String"=w314) -> ()  [unwired: 7 in, 2 out]
        n118 = disable-structure shown="Disabled" {
          disable-tunnel: [w318 "API2 Response"] -> w313
          frame Disabled {
            # "pack variant to hexstr \nif complex response is needed."
            # "complex Response"
            n119 = call "CSM - Convert Data to HexStr.vi"() -> ("HEX String (0-9,A-F)"=w318:string)  [unwired: 9 in]
          }
          frame Enabled {
          }
        }
      }
      frame "---------- Action ----------" {
        # "#CSM \"Category Seperator\"\nDo not put any code in this frame."
        n120 = call <vilib>:"Add State(s) to Queue__JKI_lib_State_Machine.vi"("State(s) in (\"\")"=w323) -> ("States Out"=w322:string)  [unwired: 14 in]
      }
      frame "Action: action1" {
        # "#CSM \"Internal State\"\nThis category is used for holding internal states"
        n121 = call <vilib>:"Add State(s) to Queue__JKI_lib_State_Machine.vi"("State(s) in (\"\")"=w327) -> ("States Out"=w326:string)  [unwired: 14 in]
      }
      frame "Action: action2" {
        # "#CSM \"Internal State\"\nThis category is used for holding internal states"
        n122 = call <vilib>:"Add State(s) to Queue__JKI_lib_State_Machine.vi"("State(s) in (\"\")"=w331) -> ("States Out"=w330:string)  [unwired: 14 in]
      }
    }
  }
